vi "7.4.vi"() -> ()   [LabVIEW 2017]
panel:
  in  "布尔":bool
  out "波形图":dbl[](graph)
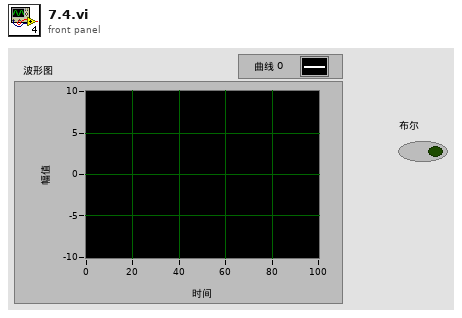
[diagram p1: front panel]
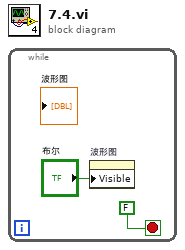
[diagram p0: block diagram]
diagram:
  n1 = while {
    stop <- FALSE stop-if-true
    n2 = property on="波形图" class="WFGraph (严格)"("Visible"="布尔") -> ()  [unwired: 2 in, 2 out]
  }
